vi "load configuration file.vi"(11 "Waveform chart":refnum<vi>) -> (3 "selected parameters":string[](array[string]))   [LabVIEW 2016]
uses:
  configuration file type def.ctl
  Communication Global variables.vi
  <vilib>/addons/_JKI.lib/Serialization/JSON/JKI JSON Serialization.lvlib
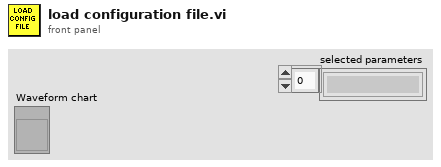
[diagram p1: front panel]
types:
  T1 = typedef "configuration file type def.ctl" = cluster{"selected parameters":string[], "REST URL":string, "UDP port":u16, "XScale.Minimum":dbl, "XScale.Maximum":dbl, "Yscale mins":dbl[], "Yscale maxs":dbl[], "Yscale colors":u32[], "LegNumRows":u32, "plot colors":u32[], "plot pointstyles":u8[], "plot names":string[], "plot yscale selections":u32[], "plot visibles":bool[]}
  T2 = enum16{"open", "replace", "create", "open or create", "replace or create", "replace or create with confirmation"}
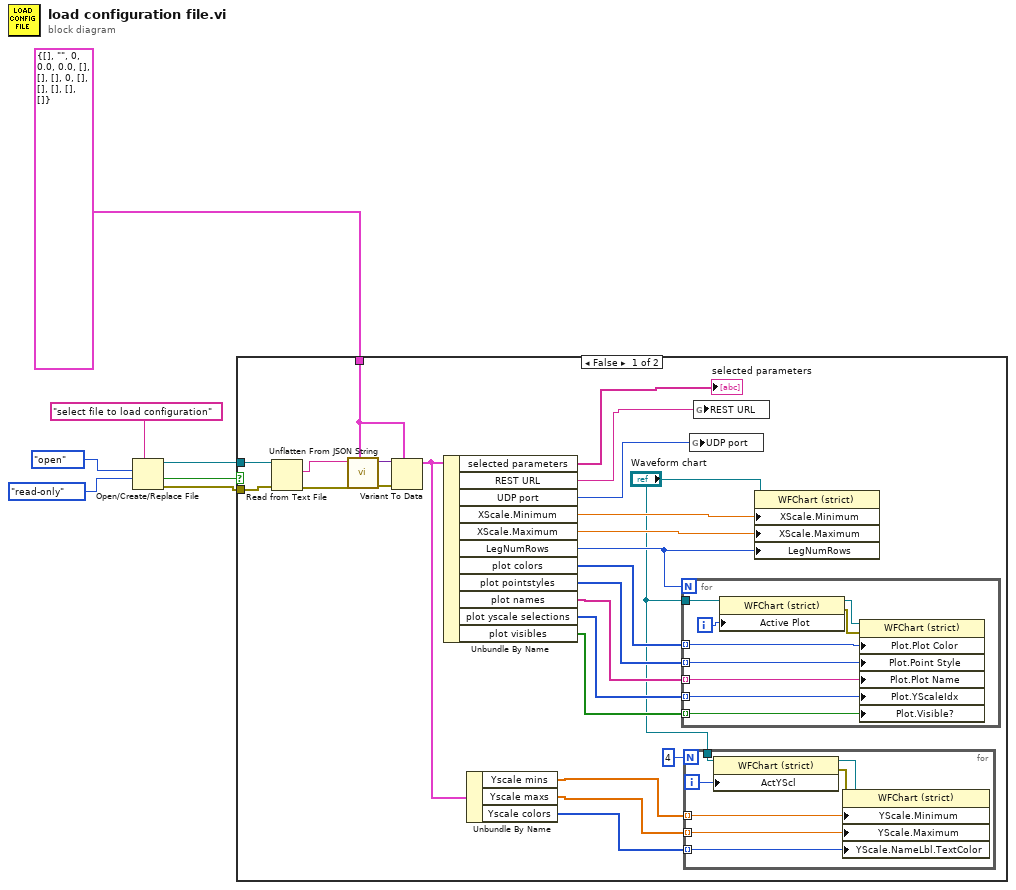
[diagram p0: block diagram]
diagram:
  n1 = Open/Create/Replace File(prompt="select file to load configuration", operation (0:open)=T2."open", access (0:read/write)=enum16{"read/write", "read-only", "write-only"}."read-only") -> (refnum out=w2:refnum<file>, cancelled=w6:bool, error out=w3:errorcluster)  [unwired: 3 in]
  n2 = case shown="False" w6 {
    tunnel: w3 -> [w31 _]
    tunnel: w2 -> [w30 _]
    tunnel: T1 {"selected parameters"=[], "REST URL"="", "UDP port"=0, "XScale.Minimum"=0.0, "XScale.Maximum"=0.0, "Yscale mins"=[], "Yscale maxs"=[], "Yscale colors"=[], "LegNumRows"=0, "plot colors"=[], "plot pointstyles"=[], "plot names"=[], "plot yscale selections"=[], "plot visibles"=[]} ("output cluster") -> [w25 _]
    frame False {
      n3 = Read from Text File(file (use dialog)=w30, error in=w31) -> (text=w29:string, error out=w28:errorcluster)  [unwired: 2 in, 2 out]
      n4 = call <vilib>:"Unflatten From JSON String.vi"("Type and Defaults"=w25, "error in (no error)"=w28, "JSON String"=w29) -> ("error out"=w27:errorcluster, "Variant"=w26:variant)  [unwired: 7 in]
      n5 = Variant To Data(error in=w27, type=w25, Variant=w26) -> (data=w13:T1)  [unwired: 1 out]
      n6 = Unbundle By Name(w13) -> ("selected parameters"=→"selected parameters":string[], "REST URL"=w23:string, "UDP port"=w22:u16, "XScale.Minimum"=w21:dbl, "XScale.Maximum"=w20:dbl, "LegNumRows"=w19:u32, "plot colors"=w18:u32[], "plot pointstyles"=w17:u8[], "plot names"=w16:string[], "plot yscale selections"=w15:u32[], "plot visibles"=w14:bool[])
      n7 = Unbundle By Name(w13) -> ("Yscale mins"=w11:dbl[], "Yscale maxs"=w10:dbl[], "Yscale colors"=w9:u32[])
      n8 = for {
        N: w19 -> [_]
        tunnel: "Waveform chart" -> [w46]
        tunnel: w18 -> [w43] mode=indexing
        tunnel: w17 -> [w42] mode=indexing
        tunnel: w16 -> [w41] mode=indexing
        tunnel: w15 -> [w40] mode=indexing
        tunnel: w14 -> [w39] mode=indexing
        i -> [w47]
        n9 = property class="WFChart (strict)"(reference=w46, "Active Plot"=w47) -> (reference out=w45:refnum<vi>, error out=w44:errorcluster)  [unwired: 1 in]
        n10 = property class="WFChart (strict)"(reference=w45, error in=w44, "Plot.Plot Color"=w43, "Plot.Point Style"=w42, "Plot.Plot Name"=w41, "Plot.YScaleIdx"=w40, "Plot.Visible?"=w39) -> ()  [unwired: 2 out]
      }
      n11 = for {
        N: 4 -> [_]
        tunnel: w11 -> [w35] mode=indexing
        tunnel: w10 -> [w34] mode=indexing
        tunnel: w9 -> [w33] mode=indexing
        tunnel: "Waveform chart" -> [w32]
        i -> [w38]
        n12 = property class="WFChart (strict)"(reference=w32, "ActYScl"=w38) -> (reference out=w37:refnum<vi>, error out=w36:errorcluster)  [unwired: 1 in]
        n13 = property class="WFChart (strict)"(reference=w37, error in=w36, "YScale.Minimum"=w35, "YScale.Maximum"=w34, "YScale.NameLbl.TextColor"=w33) -> ()  [unwired: 2 out]
      }
      n14 = global write "Communication Global variables.vi" "UDP port"(w22) -> ()
      n15 = global write "Communication Global variables.vi" "REST URL"(w23) -> ()
      n16 = property class="WFChart (strict)"(reference="Waveform chart", "XScale.Minimum"=w21, "XScale.Maximum"=w20, "LegNumRows"=w19) -> ()  [unwired: 1 in, 2 out]
    }
    frame True {
      # "cancelled"
    }
  }
